vi "graph temp and power.vi"(0 "Temperature Graph":refnum<vi>, 7 "T cont":T1 {"utility"."therm volt" format="%_6g"; "utility"."heat volt in" format="%_6g"; "utility"."heat volt out" format="%_6g"; "utility"."power out" format="%_6g"; "utility"."H Vmax" format="%_6g"; "exec"."man power" format="%_6g"; "T status"."Power" format="%_6g"; "T status"."Temp" format="%_6g"}) -> (2 "meas index":i32, 8 "T and P graph":cluster{"t hist":dbl[], "T hist":dbl[]}[](array[cluster]), 13 "T status.Temp":dbl, 14 "T status.Power":dbl)   [LabVIEW 2019]
doc: "This subVI manages the data extraction for the time, temperature, and power for the full history graph in the bug experiment. It scales the normalized power to the given temperature scale of the graph dynamically.\n\nPaul K Dixon\nP3600\nCSUSB Physics"
uses:
  typedefs/temp cont cluster.ctl
  typedefs/temp exec cluster.ctl
  typedefs/temp mode enum.ctl
  typedefs/temp indicator.ctl
  typedefs/temp cont utility.ctl
panel:
  out "P plot":cluster{"t hist":dbl[], dbl[]}
  out "T plot":cluster{"t hist":dbl[], "T hist":dbl[]}
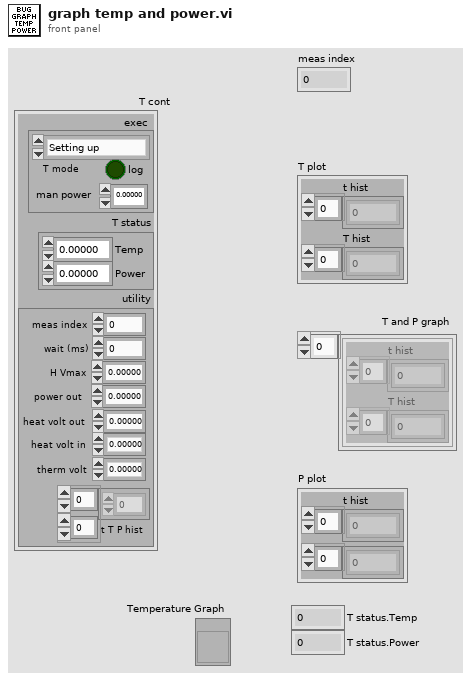
[diagram p1: front panel]
types:
  T1 = typedef "temp cont cluster.ctl" = cluster{"exec":T2, "T status":T4, "utility":T5}
  T2 = typedef "temp exec cluster.ctl" = cluster{"T mode":T3, "man power":dbl, "log":bool}
  T3 = typedef "temp mode enum.ctl" = enum16{"Setting up", "Listening to exec", "Exit"}
  T4 = typedef "temp indicator.ctl" = cluster{"Temp":dbl, "Power":dbl}
  T5 = typedef "temp cont utility.ctl" = cluster{"meas index":i32, "wait (ms)":i32, "H Vmax":dbl, "power out":dbl, "heat volt out":dbl, "heat volt in":dbl, "therm volt":dbl, "t T P hist":dbl[][]}
  T6 = cluster{"t T P hist":dbl[], "t T P hist":dbl[]}[]
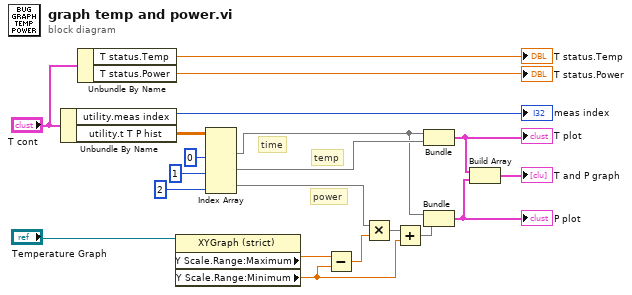
[diagram p0: block diagram]
diagram:
  # "power"
  # "temp"
  # "time"
  n1 = Unbundle By Name("T cont") -> ("utility.meas index"=→"meas index":i32, "utility.t T P hist"=w14:dbl[][])
  n2 = Unbundle By Name("T cont") -> ("T status.Temp"=→"T status.Temp":dbl, "T status.Power"=→"T status.Power":dbl)
  n3 = property class="XYGraph (strict)"(reference="Temperature Graph") -> ("Y Scale.Range:Maximum"=w20:dbl, "Y Scale.Range:Minimum"=w19:dbl)  [unwired: 1 in, 2 out]
  n4 = Index Array(array=w14, index (col) #1=0 ("disabled index (col)"), index (col) #2=1 ("index (col)"), index (col) #3=2 ("index (col)")) -> (element #1=w11:dbl[], element #2=w13:dbl[], element #3=w12:dbl[])  [unwired: 3 in]
  n5 = Subtract(x=w20, y=w19) -> (x-y=w17:dbl)
  n6 = Multiply(x=w12, y=w17) -> (x*y=w18:dbl[])
  n7 = Add(x=w18, y=w19) -> (x+y=w16:dbl[])
  n8 = Bundle("t T P hist"=w11, "t T P hist"=w13) -> (w9:cluster{"t T P hist":dbl[], "t T P hist":dbl[]})  [unwired: 1 in]
  "T plot" <- w9
  n9 = Bundle("t T P hist"=w11, w16) -> (w8:cluster{"t T P hist":dbl[], dbl[]})  [unwired: 1 in]
  "P plot" <- w8
  n10 = Build Array(w9, w8) -> (→"T and P graph":T6)
